vi "libssh2_agent_free.vi"(8 "error in (no error)":errorcluster, 11 "agent":T1) -> (0 "error out":errorcluster)   [LabVIEW 2013, in "libssh2.lvlib"]
doc: "Release memory associated with an SSH agent handle."
uses:
  libssh2.lvlib
  Agent Refnum.ctl
  Global Settings.vi
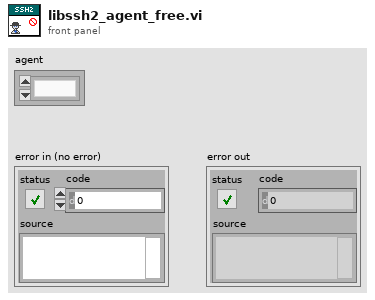
[diagram p1: front panel]
types:
  T1 = typedef "libssh2.lvlib/Agent Refnum.ctl" = refnum<k1>
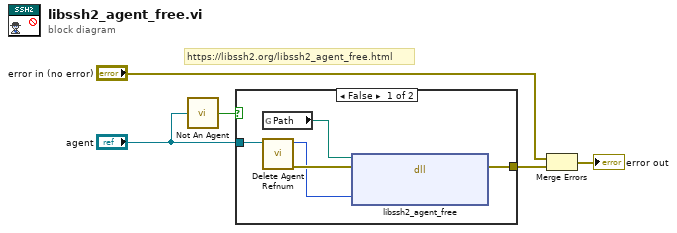
[diagram p0: block diagram]
diagram:
  # "https://libssh2.org/libssh2_agent_free.html"
  n1 = call "Not An Agent.vi"("agent"="agent") -> ("Not a Agent?"=w3:bool)
  n2 = case shown="False" w3 {
    tunnel: [w10 _] -> w5
    tunnel: "agent" -> [w6 _]
    frame False {
      n3 = global read "Global Settings.vi" "Path"() -> (w9:path)
      n4 = call "Delete Agent Refnum.vi"("agent"=w6) -> ("error out"=w8:errorcluster, "LIBSSH2_AGENT*"=w7:u64)  [unwired: 9 in]
      n5 = dll-call lib="?" fn="libssh2_agent_free"(path in=w9, error in=w8, "agent"=w7) -> (error out=w10:errorcluster)  [unwired: 3 in, 1 out]
    }
    frame True {
    }
  }
  n6 = Merge Errors("error in (no error)", w5) -> (→"error out":errorcluster)
